vi "SaveTIFF.vi"(7 "Type of scan":T1(ring)=enum."M scan", 9 "File Name":string, 10 "Data In":u8[][](array[numeric]), 11 "Current Plane":i32) -> ()   [LabVIEW 2022 SP3]
uses:
  Motion Controllers/-MotionRoutines/MotionGlobals.vi
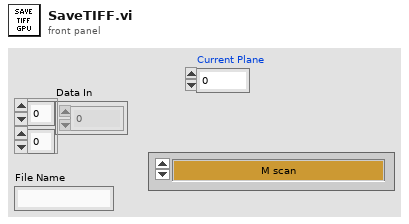
[diagram p1: front panel]
types:
  T1 = enum16{"Therapy With Scan", "M scan", "M Scan With Therapy Burst", "1-D B Scan", "1-D B Scan With Therapy Burst", "2-D B Scan", "2-D B Scan With Therapy Burst", "Rotational Scan", "1-D B-Scan PRF", "2-D B-Scan PRF", "Real-Time Scan", "Contrast Agents", "1-D w/ Real-Time Set Up", "Dual Transducer"}
  T2 = typedef "Image Type" = u32
  T3 = typedef "IMAQ Image.ctl" = refnum<image>
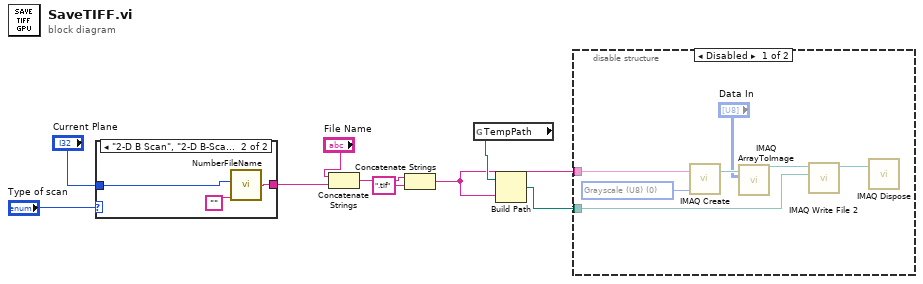
[diagram p0: block diagram]
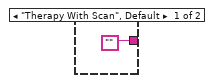
[diagram p3: hidden frame]
diagram:
  n1 = case shown="\"2-D B Scan\", \"2-D B-Scan PRF\", \"Contrast Agents\"" "Type of scan" {
    tunnel: "Current Plane" -> [_ w13]
    tunnel: ["" w11] -> w4
    frame "Therapy With Scan", Default {
    }
    frame "2-D B Scan", "2-D B-Scan PRF", "Contrast Agents" {
      n2 = call "NumberFileName.vi"("String"="", "File number"=w13) -> ("Numbered File"=w11:string)  [unwired: 2 in]
    }
  }
  n3 = Concatenate Strings("File Name", w4) -> (w1:string)
  n4 = Concatenate Strings(w1, ".tif" ("string")) -> (w6:string)
  n5 = global read "MotionGlobals.vi" "TempPath"() -> (w9:path)
  n6 = Build Path(base path=w9, name or relative path=w6) -> (appended path=w8:path)
  n7 = disable-structure shown="Disabled" {
    disable-tunnel: w8 -> [w16 _]
    disable-tunnel: w6 -> [w15 _]
    frame Disabled {
      w20 = T2 0 items=["Grayscale (U8)", "Grayscale (I16)", "Grayscale (SGL)", "Complex (CSG)", "RGB (U32)", "HSL (U32)", "RGB (U64)", "Grayscale (U16)"] ("Image Type")
      n8 = call "IMAQ Create"("Image Name"=w15, "Image Type"=w20) -> ("New Image"=w17:T3)  [unwired: 3 in, 1 out]
      n9 = call "IMAQ ArrayToImage"("Image Pixels (U8)"="Data In", "Image"=w17) -> ("Image Out"=w18:T3)  [unwired: 8 in, 1 out]
      n10 = call-poly "IMAQ Write File 2"("File Path"=w16, "Image"=w18) -> ("Image Out (duplicate)"=w19:T3)  [unwired: 8 in, 1 out]
      n11 = call "IMAQ Dispose"("Image"=w19) -> ()  [unwired: 5 in, 1 out]
    }
    frame Enabled {
    }
  }
